vi "Open Instrument.vi"(8 "error in (no error)":errorcluster, 11 "instrument.Cryostation in":refnum<class "instrument.Cryostation.lvclass">) -> (0 "error out":errorcluster, 3 "instrument.Cryostation out":refnum<class "instrument.Cryostation.lvclass">)   [LabVIEW 2019, in "instrument.Cryostation.lvclass"]
uses:
  instrument.Cryostation.lvclass
  C:/Program Files (x86)/National Instruments/LabVIEW 2019/user.lib/LevyLab/Levylab Instruments/SMOs/Instrument/Instrument.lvclass
  <userlib>/LevyLab/Levylab Instruments/SMOs/Instrument/Instrument.lvclass/Instrument.ctl
  instrument.Cryostation.lvclass/instrument.Cryostation.ctl
  <userlib>/LevyLab/Levylab Instruments/SMOs/Instrument/Instrument.lvclass
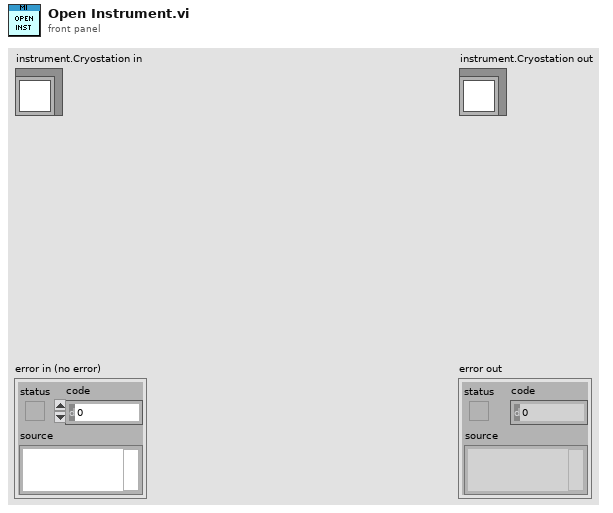
[diagram p1: front panel]
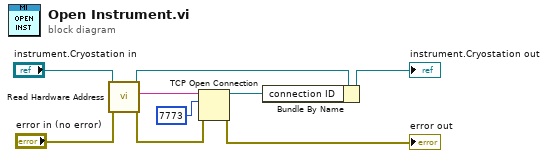
[diagram p0: block diagram]
diagram:
  n1 = call <userlib>:"Read Hardware Address.vi"("error in (no error)"="error in (no error)", "Instrument in"="instrument.Cryostation in") -> ("error out"=w6:errorcluster, "Address"=w2:string, "Instrument out"=w4:refnum<class "instrument.Cryostation.lvclass">)  [unwired: 7 in]
  n2 = TCP Open Connection(address=w2, remote port or service name=u16 7773, error in (no error)=w6) -> (connection ID=w1:refnum<k5>, error out=→"error out":errorcluster)  [unwired: 2 in]
  n3 = Bundle By Name(cluster=w4, "connection ID"=w1) -> (→"instrument.Cryostation out":refnum<class "instrument.Cryostation.lvclass">)
